vi "Load-configuration.vi"(8 "error in (no error)":errorcluster, 11 "Object ref in":T1) -> (0 "error out":errorcluster, 3 "Object ref out":T1)   [LabVIEW 2013, in "SLMControl.lvlib" / "SC-Main.lvclass"]
uses:
  SC-Main.lvclass
  Object-reference.ctl
  SC-Main.lvclass/SC-Main.ctl
  UI/Control-names.ctl
  Configuration-data.ctl
  Application-status.ctl
  Read UI.vi
  Read Status.vi
  Read Base path.vi
  <vilib>/Utility/xml.llb/Read From XML File(string).vi
  UI/Set-control-boolean.vi
  UI/Set-control-enable-single.vi
  UI/SC-UI.lvclass
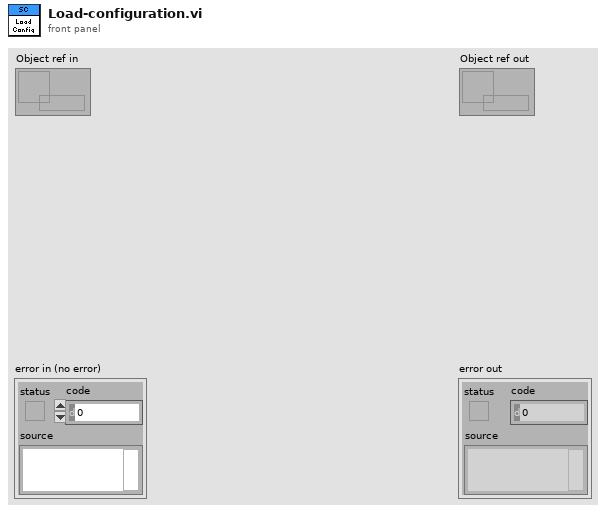
[diagram p1: front panel]
types:
  T1 = typedef "SLMControl.lvlib/SC-Main.lvclass/Object-reference.ctl" = refnum<data-value>
  T2 = typedef "SLMControl.lvlib/SC-Main.lvclass/Configuration-data.ctl" = cluster{"Deposition files":path[], "Lasing files":path[]}
  T3 = typedef "SLMControl.lvlib/SC-UI.lvclass/Control-names.ctl" = enum16{"Com-in", "Com-out", "Help", "Status", "Load configuration", "Save configuration", "Load lasing files", "Load deposition files", "Clear", "Files", "Activate", "Execute", "Abort", "Options", "Current layer", "Current iteration", "Last elapsed time", "Deposition status", "Lasing job", "Status LEDs", "Exiting led", "Initialized led", "Files loaded led", "Activated led", "Executing led", "Deposition led", "Lasing job led", "Lasing led"}
  T4 = typedef "SLMControl.lvlib/SC-Main.lvclass/Application-status.ctl" = enum16{"Idle", "Initialized", "Configured", "Activated", "Started", "Paused", "Stopped", "Reset", "Error", "Exited"}
  T5 = typedef "SLMControl.lvlib/SC-UI.lvclass/Panes-reference.ctl" = refnum<data-value>
  T6 = typedef "SLMControl.lvlib/SC-Main.lvclass/Client-status.ctl" = enum16{"Idle", "Initialized", "Configured", "Activated", "Started", "Paused", "Stopped", "Reset", "Error", "Exited"}
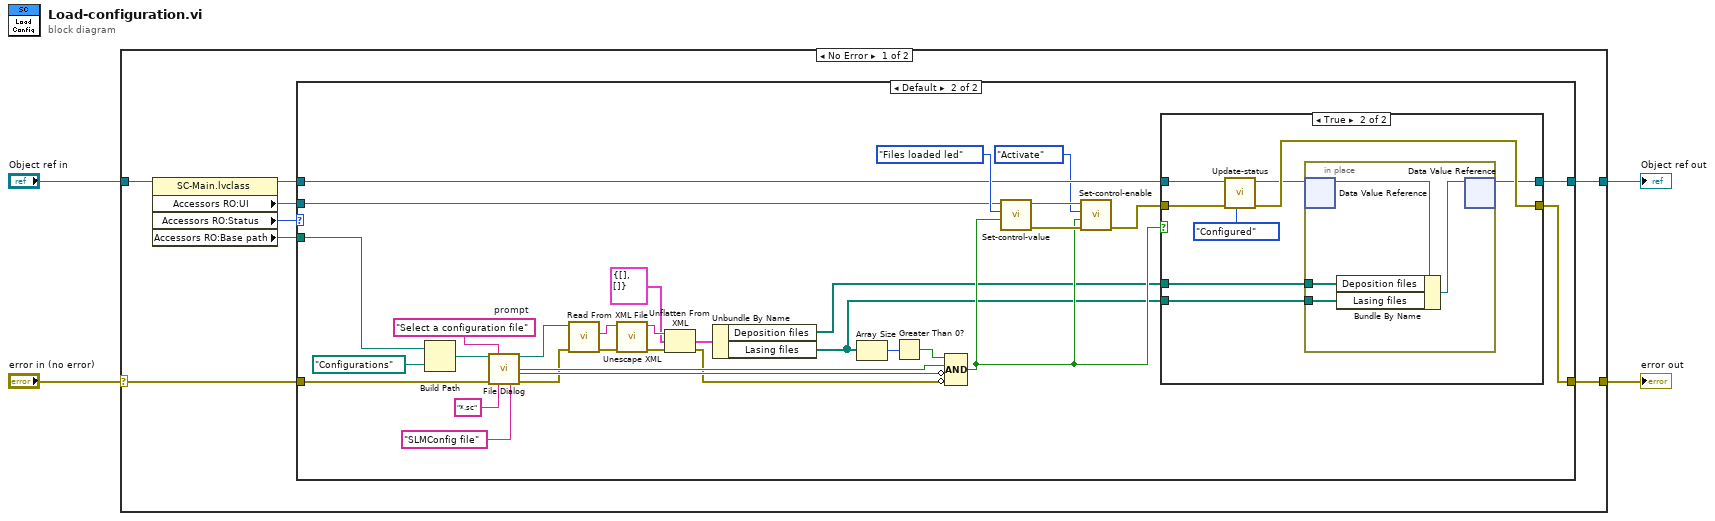
[diagram p0: block diagram]
diagram:
  n1 = case shown="No Error" "error in (no error)" {
    selector: "error in (no error)" -> [w12 w62]
    tunnel: [w8 w62] -> w3
    tunnel: [w7 w61] -> w1
    tunnel: "Object ref in" -> [w11 w61]
    frame No Error {
      n2 = property class="SC-Main.lvclass"(reference=w11) -> (reference out=w9:T1, "Accessors RO:UI"=w10:T5, "Accessors RO:Status"=w6:T6, "Accessors RO:Base path"=w5:path)  [unwired: 1 in, 1 out]
      n3 = case shown="Default" w6 {
        tunnel: w12 -> [w14 w44]
        tunnel: w10 -> [_ w37]
        tunnel: w9 -> [w13 w32]
        tunnel: [w14 w31] -> w8
        tunnel: [w13 w19] -> w7
        tunnel: w5 -> [_ w16]
        frame "Activated".."Paused" {
        }
        frame Default {
          w46 = "Select a configuration file"  # prompt
          n4 = Build Path(base path=w16, name or relative path=path "Configurations") -> (appended path=w15:path)
          n5 = call "File Dialog"("start path"=w15, "prompt"=w46, "error in"=w44, "pattern (all files)"="*.sc", "pattern label"="SLMConfig file") -> ("selected path"=w29:path, "exists"=w40:bool, "cancelled"=w39:bool, "error out"=w23:errorcluster)  [unwired: 7 in]
          n6 = call-poly <vilib>:"Read From XML File.vi"("error in (no error)"=w23, "XML File Path"=w29) -> ("error out"=w28:errorcluster, "XML Elements"=w27:string)  [unwired: 7 in, 1 out]
          n7 = call <vilib>:"Unescape XML.vi"("error in (no error)"=w28, "XML String In"=w27) -> ("error out"=w26:errorcluster, "XML String Out"=w25:string)  [unwired: 8 in]
          n8 = Unflatten From XML(xml string=w25, type=T2 {"Deposition files"=[], "Lasing files"=[]} ("Configuration data"), error in (no error)=w26) -> (value=w21:T2, error out=w22:errorcluster)
          n9 = Unbundle By Name(w21) -> ("Deposition files"=w20:path[], "Lasing files"=w18:path[])
          n10 = Array Size(array=w18) -> (size(s)=w42:i32)
          n11 = Greater Than 0?(x=w42) -> (x > 0?=w41:bool)
          n12 = Compound Arithmetic op=AND(w41, w40, invert w39, invert w22) -> (w34:bool)
          n13 = call-poly "Set-control-value.vi"("Value"=w34, "Control name"=Control-names."Files loaded led", "Panes in"=w37) -> ("error out"=w36:errorcluster, "Panes out"=w35:T5)  [unwired: 7 in]
          n14 = call-poly "Set-control-enable.vi"("error in (no error)"=w36, "Enable?"=w34, "Control name"=Control-names."Activate", "Panes in"=w35) -> ("error out"=w33:errorcluster)  [unwired: 6 in, 1 out]
          n15 = case shown="True" w34 {
            tunnel: [w47 w56] -> w31
            tunnel: [w48 w51] -> w19
            tunnel: w33 -> [w47 w53]
            tunnel: w32 -> [w48 w54]
            tunnel: w20 -> [_ w50]
            tunnel: w18 -> [_ w49]
            frame False {
            }
            frame True {
              n16 = call "Update-status.vi"("Status"=Application-status."Configured", "error in (no error)"=w53, "Object ref in"=w54) -> ("error out"=w56:errorcluster, "Object ref out"=w52:T1)  [unwired: 7 in]
              n17 = in-place {
                in-place-border: w50 -> [w58]
                in-place-border: w49 -> [w57]
                n18 = in-place-dvr #1(w52) -> (w60:refnum<class "SC-Main.lvclass">)  [unwired: 1 out]
                n19 = Bundle By Name(cluster=w60, "Deposition files"=w58, "Lasing files"=w57) -> (w59:refnum<class "SC-Main.lvclass">)
                n20 = in-place-dvr #1(w59) -> (w51:T1)  [unwired: 1 out]
              }
            }
          }
        }
      }
    }
    frame Error {
    }
  }
  "error out" <- w3
  "Object ref out" <- w1
